vi "Get Plot Scale.vi"(7 "target Domain":refnum<class "NI_Domain.lvclass">, 8 "error in (no error)":errorcluster, 11 "PDE in":refnum<class "NI_PDE.lvclass">) -> (0 "error out":errorcluster, 1 "Y Scale":T1, 2 "X Scale":T1, 3 "PDE out":refnum<class "NI_PDE.lvclass">, 4 "# of t-points":i32)   [LabVIEW 2017, in "NI_PDE.lvlib" / "NI_PDE.lvclass"]
uses:
  <vilib>/gmath/pde.llb/PDEClass/NI_PDE.lvclass
  <vilib>/Utility/miscctls.llb/LVOffsetAndMultiplierTypeDef.ctl
  <vilib>/gmath/pde.llb/DomainClass/NI_Domain.lvclass
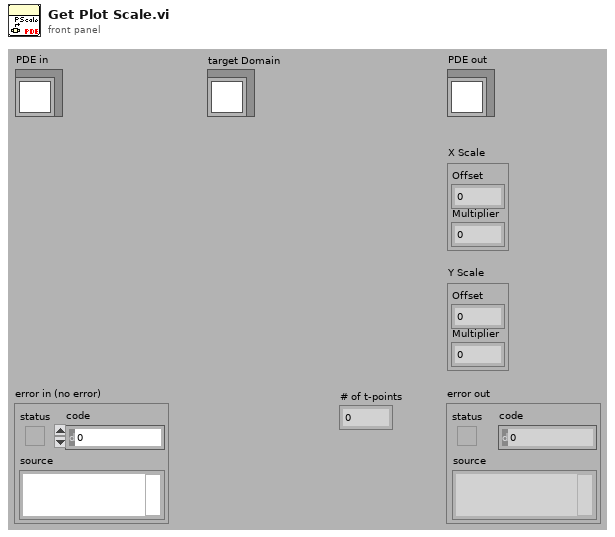
[diagram p1: front panel]
types:
  T1 = typedef "LVOffsetAndMultiplierTypeDef.ctl" = cluster{"Offset":dbl, "Multiplier":dbl}
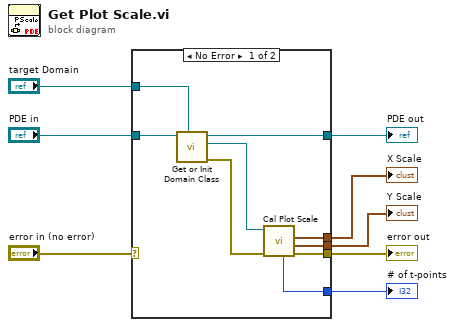
[diagram p0: block diagram]
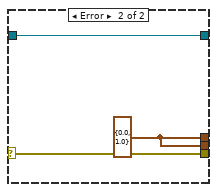
[diagram p2: hidden frame]
diagram:
  n1 = case shown="No Error" "error in (no error)" {
    selector: "error in (no error)" -> [_ w19]
    tunnel: [w13 w19] -> w8
    tunnel: "PDE in" -> [w17 w20]
    tunnel: [w16 w20] -> w6
    tunnel: "target Domain" -> [w15 _]
    tunnel: [w11 w18] -> w3
    tunnel: [w10 w18] -> w2
    tunnel: [w9 _] -> w1
    frame No Error {
      n2 = call <vilib>:"Get or Init Domain Class.vi"("target Domain"=w15, "PDE out"=w17) -> ("error out"=w14:errorcluster, "Domain out"=w12:refnum<class "NI_Domain.lvclass">, "PDE in"=w16:refnum<class "NI_PDE.lvclass">)  [unwired: 1 in, 6 out]
      n3 = call-dynamic "Cal Plot Scale.vi"("error in (no error)"=w14, "Domain in"=w12) -> ("error out"=w13:errorcluster, "Y Scale"=w10:T1, "X Scale"=w11:T1, "# of t-points"=w9:i32)  [unwired: 6 out]
    }
    frame Error {
      w18 = T1 {"Offset"=0.0, "Multiplier"=1.0} ("X Scale")
    }
  }
  "error out" <- w8
  "PDE out" <- w6
  "X Scale" <- w3
  "Y Scale" <- w2
  "# of t-points" <- w1
